vi "Package Version Constant.vi"() -> (3 "package_version":string)   [LabVIEW 2013, in "NATS Core.lvlib"]
doc: "Version of the package last built by VI Package Manager. The constant in this VI is automatically updated by the package builder's Pre-Build VI."
uses:
  NATS Core.lvlib
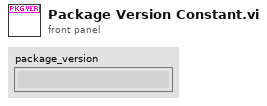
[diagram p1: front panel]
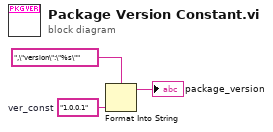
[diagram p0: block diagram]
diagram:
  w2 = "1.0.0.1"  # ver_const
  n1 = Format Into String(format string=",\"version\":\"%s\"", w2) -> (resulting string=→"package_version":string)  [unwired: 2 in, 1 out]
